vi "Meas Write Record Header File.vi"(6 "samples count":i64, 7 "corrections":T1 {"transducers"."channels"."Phase index" min=1 step=1}, 8 "error in":errorcluster, 9 "adc session":T4={"niScope"={"channel cfg"=[], "sessions"=[], "multi cards"=FALSE, "channels"=0, "type"=enum."n/a", "memory [B/chn]"=0, "ext. clock [Hz]"=0.0, "samples count"=0, "use streaming"=FALSE, "proc setup"={"packet size [smpl]"=0, "current timeout [s]"=0.0, "blk2blk timeout [s]"=0.0, "event time"=timestamp(0 s since 1904-01-01), "temp sampl T [s]"=0.0, "data queue"=refnum, "stop notifier"=refnum, "proc ref"=refnum}, "sample width [B]"=0, "ranges [V]"=[], "trigger setup"={"coupling"=1, "level [V]"=0.0, "slope"=0, "mode"=enum."Immediate"}, "fs [Hz]"=0.0, "bitres [bit]"=0}, "3458A"={"channels"=[], "sync unit"={"VISA"="", "type"=enum."Picotest U6200A"}, "awg unit"={"type"=enum."Agilent 331xxA to 332xxA", "VISA"="", "enable 10MHz ref"=FALSE}, "sync mode"=enum."MASTER-SLAVE, MASTER clocked by TIMER", "streaming mode"=FALSE, "idn mode"=enum."Auto", "sampling mode"=enum."DCV", "Ts [s]"=0.0, "sample memory [B]"=0, "proc setup"={"channel id"=0, "packet size [smpl]"=0, "current timeout [s]"=0.0, "blk2blk timeout [s]"=0.0, "event time"=timestamp(0 s since 1904-01-01), "stop notifier"=refnum, "data queues"=[], "proc refs"=[], "bus semaphore"=refnum}, "sample size [B]"=0, "sample count"=0, "aux data"={"channel id"=0, "valid?"=[], "gain [V]"=[], "timestamp [s]"=[], "Ts [s]"=0.0, "abs timestamp"=timestamp(0 s since 1904-01-01), "t [deg C]"=[]}, "ranges [V]"=[], "aperture [s]"=0.0, "LEVEL trigger"={"edge"=enum."POS", "level [V]"=0.0, "coupling"=enum."DC"}, "trigger mode"=enum."AUTO", "measure temp.?"=FALSE, "disp mesages"=[], "shared bus?"=FALSE, "disable display?"=FALSE, "aper mode"=enum."Manual", "aper rules"=[]}, "dsdll"={"dsdll"={"dsdll path"=path "", "dsdll handle"=[], "output devices"=[], "capture devices"=[]}, "channels"=0, "device id"=0, "channel idns"=[], "proc setup"={"packet size [smpl]"=0, "current timeout [s]"=0.0, "blk2blk timeout [s]"=0.0, "event time"=timestamp(0 s since 1904-01-01), "data queue"=refnum, "stop notifier"=refnum, "proc ref"=refnum}, "samples count"=0, "fs [Hz]"=0.0}, "type"=enum."niScope", "channel idn str"=[], "aux instr idn str"=[], "modified?"=FALSE, "simadc"={"channels"=[], "range [V]"=0.0, "Ts step [s]"=0.0, "time [s]"=0.0, "fs [Hz]"=0.0, "count"=0, "smpl offset"=0, "set count"=0, "bit res"=0}, "force rst?"=FALSE, "exit mode"=enum."Immediate reset", "exit dly"=0.0, "exit tmr"=timestamp(0 s since 1904-01-01), "busy?"=FALSE, "accessed?"=FALSE, "QuADC session"={"channel cfg"=[], "sessions"=[], "multi cards"=FALSE, "channels"=0, "type"=enum."n/a", "memory [B/chn]"=0, "ext. clock [Hz]"=0.0, "samples count"=0, "use streaming"=FALSE, "proc setup"={"packet size [smpl]"=0, "current timeout [s]"=0.0, "blk2blk timeout [s]"=0.0, "event time"=timestamp(0 s since 1904-01-01), "temp sampl T [s]"=0.0, "data queue"=refnum, "stop notifier"=refnum, "proc ref"=refnum}, "sample width [B]"=0, "ranges [V]"=[], "trigger setup"={"coupling"=1, "level [V]"=0.0, "slope"=0, "mode"=enum."Immediate"}, "fs [Hz]"=0.0, "bitres [bit]"=0}} {"QuADC session"."trigger setup"."level [V]" format="%.2f"; "QuADC session"."trigger setup"."coupling" items=["AC"=0, "DC"=1, "HF Reject"=3, "LF Reject"=4, "AC Plus HF Reject"=1001]; "QuADC session"."channel cfg"."Clock fr. (Hz)" min=0.0 format="%#_9p"; "QuADC session"."channel cfg"."Number of JJ" min=1; "QuADC session"."channel cfg"."Range [Vpk]" min=0.0; "QuADC session"."channel cfg"."Channel" min=0; "3458A"."channels"."Range [Vpk]" min=0.0; "niScope"."trigger setup"."level [V]" format="%.2f"; "niScope"."trigger setup"."coupling" items=["AC"=0, "DC"=1, "HF Reject"=3, "LF Reject"=4, "AC Plus HF Reject"=1001]; "niScope"."channel cfg"."Range [Vpk]" min=0.0; "niScope"."channel cfg"."Channel" min=0}, 10 "aux data":T53, 11 "sequence item":T49) -> (0 "error out":errorcluster)   [LabVIEW 2013]
doc: "Write logged temperature data to the samples MAT file. It will write the data even if they are empty."
uses:
  adc/ADC Aux Data.ctl
  Meas Sequence Item.ctl
  Meas Sampling Configuration.ctl
  adc/ADC Trig Config.ctl
  adc/ADC Trig Mode Source.ctl
  adc/ADC Trig Coupling.ctl
  adc/ADC Trig Slope.ctl
  processing/QWTB/Meas Proc QWTB Algorithm Parameter Data.ctl
  adc/ADC Session.ctl
  drivers/niScope/niScope Session.ctl
  drivers/niScope/niScope Virtual Channel Config.ctl
  drivers/niScope/niScope Virtual Channel Mode.ctl
  drivers/niScope/niScope Virtual Channel Input Z.ctl
  drivers/niScope/niScope Virtual Channel Coupling.ctl
  drivers/niScope/niScope Type.ctl
  drivers/niScope/niScope Digitizing Process Options.ctl
  drivers/niScope/niScope Data Packet.ctl
  drivers/niScope/niScope Trigger Setup.ctl
  <instrlib>/niScope/Controls/niScope trigger coupling.ctl
  <instrlib>/niScope/Controls/niScope trigger slope.ctl
  drivers/DMM/3458A Digitizer Session.ctl
  drivers/DMM/3458A Virtual Channel Config.ctl
  drivers/Counter/Counter Session.ctl
  drivers/Counter/Counter Type.ctl
  drivers/AWG/AWG Session.ctl
  drivers/AWG/AWG Type.ctl
  drivers/DMM/3458A Sync Mode.ctl
  drivers/DMM/3458A Idn Mode.ctl
  drivers/DMM/3458A Digitizing Low Levels/Configure/Sampling Mode.ctl
  drivers/DMM/3458A Digitizing Process Options.ctl
  drivers/DMM/3458A Data Packet.ctl
  drivers/DMM/3458A Aux Record Data.ctl
  drivers/DMM/3458A Digitizing Low Levels/Configure/Level Setup.ctl
  drivers/DMM/3458A Digitizing Low Levels/Configure/First Sample Trigger.ctl
  drivers/DMM/3458A Aperture Selection Mode.ctl
  drivers/dsdll/DSDLL Session.ctl
  drivers/dsdll/dsdll.lvlibp/dsdll_instance.ctl
  drivers/dsdll/dsdll.lvlibp/dsdll_device_record.ctl
  drivers/dsdll/DSDLL Process Config.ctl
  drivers/dsdll/DSDLL Data Packet.ctl
  adc/ADC Type.ctl
  drivers/simulated_adc/SimAdc Config.ctl
  drivers/simulated_adc/SimAdc Channel Cfg.ctl
  adc/ADC On Close Action.ctl
  drivers/Quatsch_driver/QuADCDriver/QuADC Session.ctl
  drivers/Quatsch_driver/QuADCDriver/QuADC Virtual Channel Config.ctl
  drivers/Quatsch_driver/QuADCDriver/QuADC Virtual Channel Mode.ctl
  drivers/Quatsch_driver/QuADCDriver/QuADC Virtual Channel Input Z.ctl
  drivers/Quatsch_driver/QuADCDriver/QuADC Virtual Channel Coupling.ctl
  drivers/Quatsch_driver/QuADCDriver/QuADC Type.ctl
  drivers/Quatsch_driver/QuADCDriver/QuADC Digitizing Process Options.ctl
  drivers/Quatsch_driver/QuADCDriver/QuADC Data Packet.ctl
  drivers/Quatsch_driver/QuADCDriver/QuADC Trigger Setup.ctl
  Corrections/Corr Setup.ctl
  Corrections/Corr Tranducer Item.ctl
  Corrections/Corr Digitizers.ctl
  <vilib>/Analysis/baseanly.llb/Mean (DBL).vi
  octave/infolib.lvlibp/Private/Add matrix polymorph parts/1D String.vi
  octave/infolib.lvlibp/Private/Add key polymorph parts/I64.vi
  octave/infolib.lvlibp/Private/Add key polymorph parts/String.vi
  octave/infolib.lvlibp/Private/Add key polymorph parts/Boolean.vi
  octave/infolib.lvlibp/Private/Get key polymorph parts/GetI64.vi
  octave/infolib.lvlibp/Private/Add key polymorph parts/EXT.vi
  octave/infolib.lvlibp/Private/Add matrix polymorph parts/2D EXT.vi
  octave/infolib.lvlibp/Private/Add matrix polymorph parts/2D String.vi
  octave/infolib.lvlibp
  <vilib>/Analysis/NI_AALBase.lvlib
  drivers/niScope/niScope Virtual Digitizer.lvlib
  drivers/DMM/3458A Virtual Digitizer.lvlib
  drivers/Counter/Counter.lvlib
  drivers/AWG/AWG.lvlib
  drivers/DMM/3458A Digitizing Low Levels/3458A Digitizing Low Levels.lvlib
  drivers/dsdll/dsdll.lvlibp
  drivers/dsdll/DSDLL Virtual Digitizer.lvlib
  drivers/Quatsch_driver/QuADCDriver/QuADC Virtual Digitizer.lvlib
panel:
  in  "coupling":T46
  in  "slope":T47
  in  "source":T48
  # "ADC:"
  # "IP Address"
  # "."
  # "."
  # "."
  # ":"
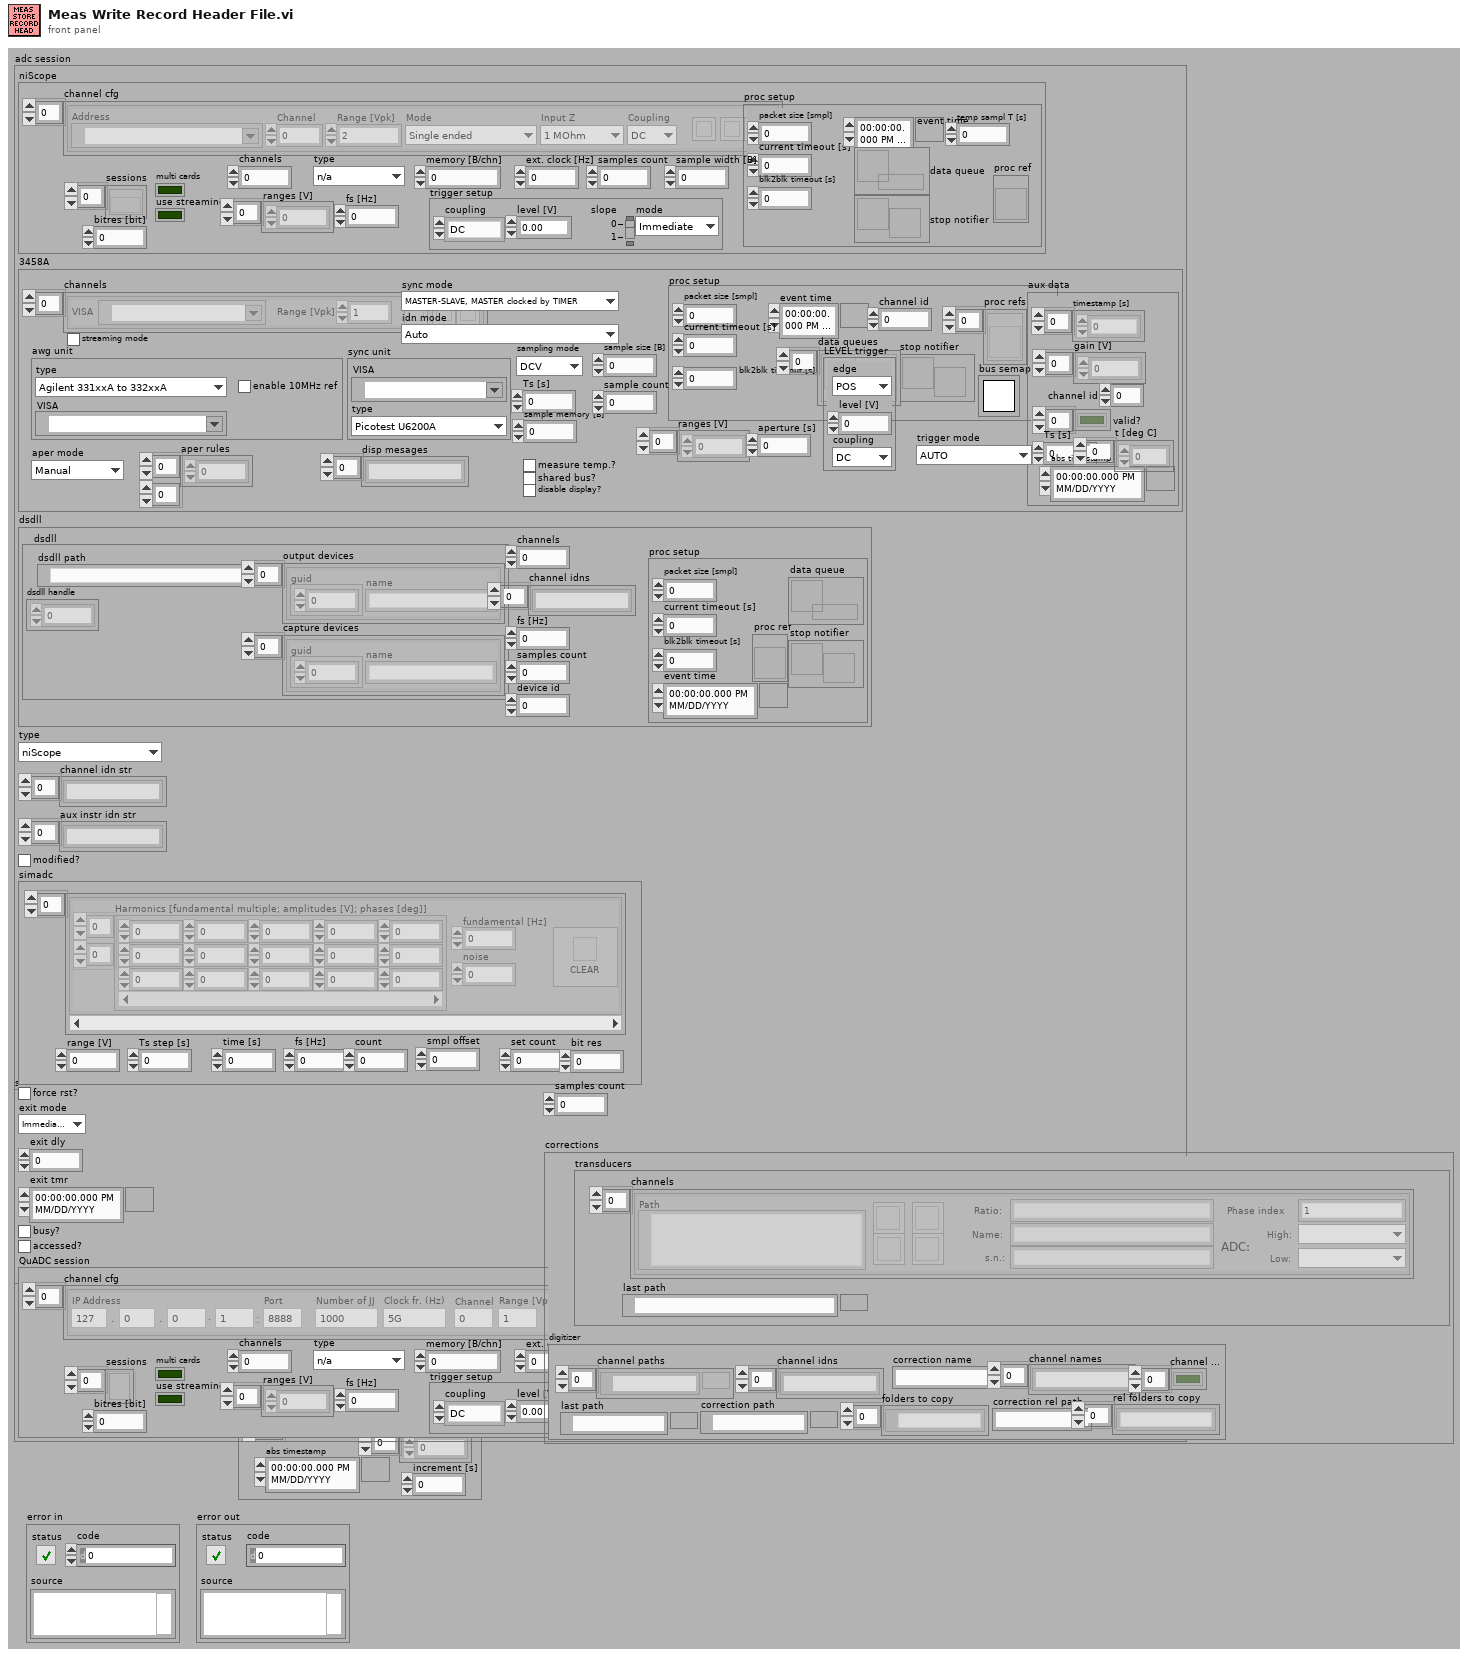
[diagram p1: front panel]
types:
  T1 = typedef "Corr Setup.ctl" = cluster{"transducers":cluster{"channels":T2[], "last path":path}, "digitizer":T3}
  T2 = typedef "Corr Tranducer Item.ctl" = cluster{"Path":path, "Ratio:":string, "Name:":string, "btn rem":bool, "btn up":bool, "btn down":bool, "s.n.:":string, "btn open":bool, "ratio o/i":dbl, "chn hi":u16, "chn lo":u16, "Phase index":i32}
  T3 = typedef "Corr Digitizers.ctl" = cluster{"last path":path, "channel paths":path[], "channel idns":string[], "correction name":string, "channel names":string[], "folders to copy":path[], "channel valid":bool[], "correction path":path, "correction rel path":string, "rel folders to copy":string[]}
  T4 = typedef "ADC Session.ctl" = cluster{"niScope":T5, "3458A":T15, "dsdll":T30, "type":T34, "channel idn str":string[], "aux instr idn str":string[], "modified?":bool, "simadc":T35, "force rst?":bool, "exit mode":T37, "exit dly":dbl, "exit tmr":timestamp, "busy?":bool, "accessed?":bool, "QuADC session":T38}
  T5 = typedef "niScope Virtual Digitizer.lvlib/niScope Session.ctl" = cluster{"channel cfg":T6[], "sessions":refnum<k20>[], "multi cards":bool, "channels":i32, "type":T10, "memory [B/chn]":i32, "ext. clock [Hz]":dbl, "samples count":i64, "use streaming":bool, "proc setup":T11, "sample width [B]":i32, "ranges [V]":dbl[], "trigger setup":T12, "fs [Hz]":dbl, "bitres [bit]":i32}
  T6 = typedef "niScope Virtual Digitizer.lvlib/niScope Virtual Channel Config.ctl" = cluster{"Address":refnum<k15>, "Channel":i32, "Mode":T7, "Input Z":T8, "Coupling":T9, "Range [Vpk]":dbl, "btn clr":bool, "btn up":bool, "btn down":bool}
  T7 = typedef "niScope Virtual Digitizer.lvlib/niScope Virtual Channel Mode.ctl" = enum16{"Single ended", "Unbal. differential", "Differential"}
  T8 = typedef "niScope Virtual Digitizer.lvlib/niScope Virtual Channel Input Z.ctl" = enum16{"1 MOhm", "50 Ohm"}
  T9 = typedef "niScope Virtual Digitizer.lvlib/niScope Virtual Channel Coupling.ctl" = enum16{"AC", "DC", "GND"}
  T10 = typedef "niScope Virtual Digitizer.lvlib/niScope Type.ctl" = enum16{"n/a", "5922"}
  T11 = typedef "niScope Virtual Digitizer.lvlib/niScope Digitizing Process Options.ctl" = cluster{"packet size [smpl]":i64, "current timeout [s]":dbl, "blk2blk timeout [s]":dbl, "event time":timestamp, "temp sampl T [s]":dbl, "data queue":refnum<queue>, "stop notifier":refnum<notifier>, "proc ref":refnum<vi>}
  T12 = typedef "niScope Virtual Digitizer.lvlib/niScope Trigger Setup.ctl" = cluster{"coupling":T13, "level [V]":dbl, "slope":T14, "mode":enum16{"Immediate", "External", "Level"}}
  T13 = typedef "niScope trigger coupling.ctl" = u16
  T14 = typedef "niScope trigger slope.ctl" = i32
  T15 = typedef "3458A Virtual Digitizer.lvlib/3458A Digitizer Session.ctl" = cluster{"channels":T16[], "sync unit":T17, "awg unit":T19, "sync mode":T21, "streaming mode":bool, "idn mode":T22, "sampling mode":T23, "Ts [s]":dbl, "sample memory [B]":i32, "proc setup":T24, "sample size [B]":i32, "sample count":i32, "aux data":T26, "ranges [V]":dbl[], "aperture [s]":dbl, "LEVEL trigger":T27, "trigger mode":T28, "measure temp.?":bool, "disp mesages":string[], "shared bus?":bool, "disable display?":bool, "aper mode":T29, "aper rules":dbl[][]}
  T16 = typedef "3458A Virtual Digitizer.lvlib/3458A Virtual Channel Config.ctl" = cluster{"VISA":refnum<visa-resource-name>, "Range [Vpk]":dbl, "btn clr":bool, "btn up":bool, "btn down":bool}
  T17 = typedef "Counter.lvlib/Counter Session.ctl" = cluster{"VISA":refnum<visa-resource-name>, "type":T18}
  T18 = typedef "Counter.lvlib/Counter Type.ctl" = enum16{"Picotest U6200A", "dummy"}
  T19 = typedef "AWG.lvlib/AWG Session.ctl" = cluster{"type":T20, "VISA":refnum<visa-resource-name>, "enable 10MHz ref":bool}
  T20 = typedef "AWG.lvlib/AWG Type.ctl" = enum16{"Agilent 331xxA to 332xxA", "Agilent 335xxA to 336xxA", "Tektronix AFG3101C", "dummy"}
  T21 = typedef "3458A Virtual Digitizer.lvlib/3458A Sync Mode.ctl" = enum16{"MASTER-SLAVE, MASTER clocked by TIMER", "MASTER-SLAVE, MASTER clocked by AWG", "ALL clocked by AWG", "MASTER-SLAVE, ALL clocked by TIMER", "ALL clocked by AWG with DFLL"}
  T22 = typedef "3458A Virtual Digitizer.lvlib/3458A Idn Mode.ctl" = enum16{"Auto", "Sequential (chn A, chn B, ...)", "From calibration string"}
  T23 = typedef "3458A Virtual Digitizer.lvlib/3458A Digitizing Low Levels.lvlib/Sampling Mode.ctl" = enum16{"DCV", "DSDC", "DSAC"}
  T24 = typedef "3458A Virtual Digitizer.lvlib/3458A Digitizing Process Options.ctl" = cluster{"channel id":i32, "packet size [smpl]":i32, "current timeout [s]":dbl, "blk2blk timeout [s]":dbl, "event time":timestamp, "stop notifier":refnum<notifier>, "data queues":refnum<queue>[], "proc refs":refnum<vi>[], "bus semaphore":T25}
  T25 = typedef "Semaphore RefNum" = refnum<k1>
  T26 = typedef "3458A Virtual Digitizer.lvlib/3458A Aux Record Data.ctl" = cluster{"channel id":i32, "valid?":bool[], "gain [V]":dbl[], "timestamp [s]":dbl[], "Ts [s]":dbl, "abs timestamp":timestamp, "t [deg C]":dbl[]}
  T27 = typedef "3458A Virtual Digitizer.lvlib/3458A Digitizing Low Levels.lvlib/Level Setup.ctl" = cluster{"edge":enum16{"POS", "NEG"}, "level [V]":dbl, "coupling":enum16{"DC", "AC"}}
  T28 = typedef "3458A Virtual Digitizer.lvlib/3458A Digitizing Low Levels.lvlib/First Sample Trigger.ctl" = enum16{"AUTO", "EXT", "SYN", "SGL", "HOLD", "LEVEL"}
  T29 = typedef "3458A Virtual Digitizer.lvlib/3458A Aperture Selection Mode.ctl" = enum16{"Manual", "Maximum", "Table"}
  T30 = typedef "DSDLL Virtual Digitizer.lvlib/DSDLL Session.ctl" = cluster{"dsdll":T31, "channels":i32, "device id":i32, "channel idns":string[], "proc setup":T33, "samples count":i32, "fs [Hz]":dbl}
  T31 = typedef "dsdll.lvlibp/dsdll_instance.ctl" = cluster{"dsdll path":path, "dsdll handle":u8[], "output devices":T32[], "capture devices":T32[]}
  T32 = typedef "dsdll.lvlibp/dsdll_device_record.ctl" = cluster{"guid":u8[], "name":string}
  T33 = typedef "DSDLL Virtual Digitizer.lvlib/DSDLL Process Config.ctl" = cluster{"packet size [smpl]":i32, "current timeout [s]":dbl, "blk2blk timeout [s]":dbl, "event time":timestamp, "data queue":refnum<queue>, "stop notifier":refnum<notifier>, "proc ref":refnum<vi>}
  T34 = typedef "ADC Type.ctl" = enum16{"niScope", "3458A", "DirectSound DLL", "dummy", "QuADC"}
  T35 = typedef "SimAdc Config.ctl" = cluster{"channels":T36[], "range [V]":dbl, "Ts step [s]":dbl, "time [s]":dbl, "fs [Hz]":dbl, "count":i64, "smpl offset":i64, "set count":i64, "bit res":i32}
  T36 = typedef "SimAdc Channel Cfg.ctl" = cluster{"harmonics":dbl[][], "btn clear":bool, "noise":dbl, "fundamental [Hz]":dbl}
  T37 = typedef "ADC On Close Action.ctl" = enum16{"Immediate reset", "Delayed reset"}
  T38 = typedef "QuADC Virtual Digitizer.lvlib/QuADC Session.ctl" = cluster{"channel cfg":T39[], "sessions":refnum<k5>[], "multi cards":bool, "channels":i32, "type":T43, "memory [B/chn]":i32, "ext. clock [Hz]":dbl, "samples count":i64, "use streaming":bool, "proc setup":T44, "sample width [B]":i32, "ranges [V]":dbl[], "trigger setup":T45, "fs [Hz]":dbl, "bitres [bit]":i32}
  T39 = typedef "QuADC Virtual Digitizer.lvlib/QuADC Virtual Channel Config.ctl" = cluster{"Channel":i32, "Mode":T40, "Input Z":T41, "Coupling":T42, "Range [Vpk]":dbl, "btn clr":bool, "btn up":bool, "btn down":bool, "IP address A":u8, "IP address B":u8, "IP address C":u8, "IP address D":u8, "Port":u16, "Number of JJ":u32, "Clock fr. (Hz)":dbl}
  T40 = typedef "QuADC Virtual Digitizer.lvlib/QuADC Virtual Channel Mode.ctl" = enum16{"Single ended", "Unbal. differential", "Differential"}
  T41 = typedef "QuADC Virtual Digitizer.lvlib/QuADC Virtual Channel Input Z.ctl" = enum16{"1 MOhm", "50 Ohm"}
  T42 = typedef "QuADC Virtual Digitizer.lvlib/QuADC Virtual Channel Coupling.ctl" = enum16{"AC", "DC", "GND"}
  T43 = typedef "QuADC Virtual Digitizer.lvlib/QuADC Type.ctl" = enum16{"n/a", "v1"}
  T44 = typedef "QuADC Virtual Digitizer.lvlib/QuADC Digitizing Process Options.ctl" = cluster{"packet size [smpl]":i64, "current timeout [s]":dbl, "blk2blk timeout [s]":dbl, "event time":timestamp, "temp sampl T [s]":dbl, "data queue":refnum<queue>, "stop notifier":refnum<notifier>, "proc ref":refnum<vi>}
  T45 = typedef "QuADC Virtual Digitizer.lvlib/QuADC Trigger Setup.ctl" = cluster{"coupling":T13, "level [V]":dbl, "slope":T14, "mode":enum16{"Immediate", "External", "Level"}}
  T46 = typedef "ADC Trig Coupling.ctl" = enum16{"DC", "AC"}
  T47 = typedef "ADC Trig Slope.ctl" = enum16{"POS", "NEG"}
  T48 = typedef "ADC Trig Mode Source.ctl" = enum16{"Immediate", "External", "Level"}
  T49 = typedef "Meas Sequence Item.ctl" = cluster{"config":T50, "data file path":path, "header file path":path, "group id":i32, "average id":i32, "group done?":bool, "adc modified?":bool, "source modified?":bool, "progress [%]":dbl, "groups cnt":i32, "average cnt":i32, "data file relative path":string, "meas root path":path, "calculate?":bool}
  T50 = typedef "Meas Sampling Configuration.ctl" = cluster{"fs [Hz]":dbl, "count [smpl]":i64, "aperture [s]":dbl, "trigger":T51, "ranges [Vpk]":dbl[], "QWTB parameters":T52[]}
  T51 = typedef "ADC Trig Config.ctl" = cluster{"source":T48, "level [V]":dbl, "coupling":T46, "slope":T47}
  T52 = typedef "Meas Proc QWTB Algorithm Parameter Data.ctl" = cluster{"name":string, "numerics":dbl[], "strings":string[]}
  T53 = typedef "ADC Aux Data.ctl" = cluster{"offset [V]":dbl[], "gain [V]":dbl[], "time stamp [s]":dbl[], "increment [s]":dbl, "T smpl":i64[], "T [deg C]":dbl[][], "valid?":bool, "abs timestamp":timestamp}
  T54 = typedef "ADC Capabilities.ctl" = cluster{"max samples count":i64, "max fs [Hz]":ext, "min fs [Hz]":ext, "Ts step [s]":ext, "max Ts [s]":ext, "min Ts [s]":ext, "allows streaming?":bool, "streaming on?":bool, "has level trig?":bool, "has ext trig?":bool, "has aperture?":bool, "aper min [s]":dbl, "aper max [s]":dbl, "channels count":i32, "has ranges?":bool, "has temperature?":bool, "has temperature log?":bool, "has selfcal?":bool, "fs step [Hz]":ext, "smpl rate step mode":T55}
  T55 = typedef "ADC Sampling Rate Step Mode.ctl" = enum16{"const period", "const frequency"}
  T56 = typedef "ADC Attribute.ctl" = cluster{"name":string, "value":string[], "is constant per group":bool}
  T57 = typedef "ADC Current Configuration.ctl" = cluster{"count [smpl]":i64, "channels count":i32, "fs [Hz]":dbl, "ranges [V]":dbl[], "trigger":T51, "ext freq. locked?":bool, "streaming on?":bool, "is int16?":bool, "bitres":i32}
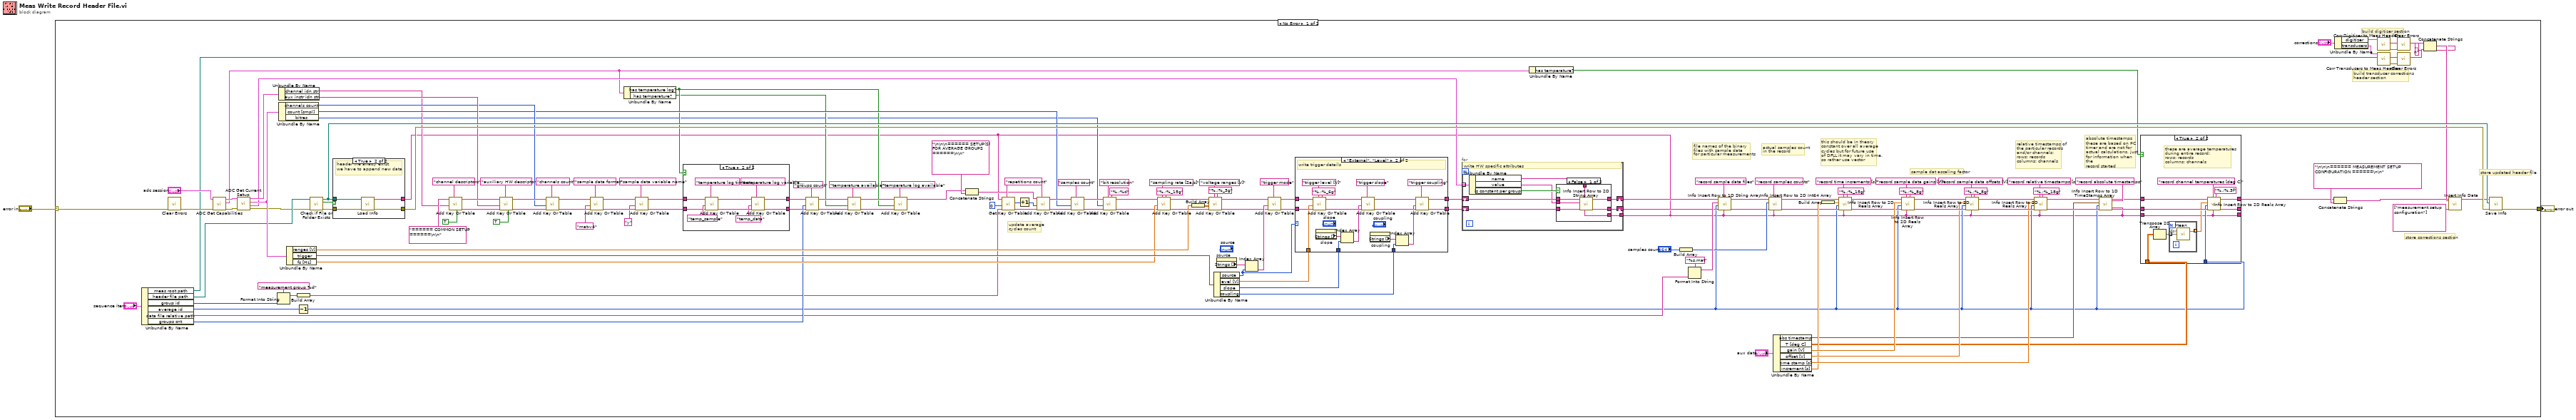
[diagram p0: block diagram]
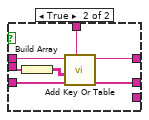
[diagram p4: hidden frame]
diagram:
  n1 = case shown="No Error" "error in" {
    selector: "error in" -> [w100 w237]
    tunnel: [w134 w237] -> w2
    frame No Error {
      w132 = "repetitions count" ("key description")
      # "store corrections section"
      # "build digitizer section"
      # "build transducer corrections\nheader section"
      # "actual samples count\nin the record"
      # "absolute timestamps\nthese are based on PC\ntimer and are not for \nactual calculations, just\nfor information when the\nrecord started"
      # "file names of the binary\nfiles with sample data\nfor particular measurements"
      # "relative timestamps of\nthe particular records\nand/or channels:\nrows: records\ncolumns: channels"
      # "sample dat ascaling factor"
      # "this should be in theory\nconstant over all average\ncycles but for future use\nof DFLL it may vary in time,\nso rather use vector"
      # "update average\ncycles count"
      # "store updated header file"
      n2 = Unbundle By Name("sequence item") -> ("meas root path"=w27:path, "header file path"=w34:path, "group id"=w47:i32, "average id"=w127:i32, "data file relative path"=w33:string, "groups cnt"=w46:i32)
      n3 = call <vilib>:"Clear Errors.vi"("error in (no error)"=w100) -> ("error out"=w76:errorcluster)  [unwired: 6 in]
      n4 = call "ADC Get Capabilities.vi"("error in"=w76, "adc session in"="adc session") -> ("error out"=w77:errorcluster, "capabilities"=w51:T54, "adc session out"=w74:T4)  [unwired: 7 in]
      n5 = call "ADC Get Current Setup.vi"("error in"=w77, "adc session in"=w74) -> ("error out"=w21:errorcluster, "device specific attributes"=w80:T56[], "common attributes"=w84:T57, "adc session out"=w110:T4)  [unwired: 6 in]
      n6 = Format Into String(format string="measurement group %d", w47) -> (resulting string=w112:string)  [unwired: 2 in, 1 out]
      n7 = Unbundle By Name(w110) -> ("channel idn str"=w14:string[], "aux instr idn str"=w106:string[])
      n8 = Unbundle By Name(w84) -> ("channels count"=w90:i32, "count [smpl]"=w58:i64, "bitres"=w5:i32)
      n9 = Unbundle By Name(w84) -> ("ranges [V]"=w83:dbl[], "trigger"=w82:T51, "fs [Hz]"=w81:dbl)
      n10 = Build Array(w112) -> (w22:string[])
      n11 = Decrement(x=w127) -> (x-1=w23:i32)
      n12 = call <vilib>:"Check if File or Folder Exists.vi"("error in (no error)"=w21, "path"=w34) -> ("error out"=w157:errorcluster, "file or folder exists?"=w158:bool, "dup path"=w136:path)  [unwired: 7 in]
      n13 = case shown="True" w158 {
        tunnel: w157 -> [w232 w236]
        tunnel: w136 -> [_ w235]
        tunnel: [_ w234] -> w4
        tunnel: [w232 w233] -> w135
        frame False {
          # "no header file exit\nstart new one"
        }
        frame True {
          # "header file alrady exist\nwe have to append new data"
          n14 = call "Load Info.vi"("error in"=w236, "filename"=w235) -> ("error out"=w233:errorcluster, "info data"=w234:string)  [unwired: 8 in]
        }
      }
      n15 = call-poly "Add Key Or Table.vi"("column vector (F)"=TRUE, "key description"="channel descriptors", "string"=w14, "info data"="====== COMMON SETUP ======\n\n" ("string")) -> ("sections out"=w109:string[], "info data out"=w108:string)  [unwired: 6 in]
      n16 = call-poly "Add Key Or Table.vi"("column vector (F)"=TRUE, "key description"="auxiliary HW descriptors", "sections"=w109, "string"=w106, "info data"=w108) -> ("sections out"=w103:string[], "info data out"=w102:string)  [unwired: 5 in]
      n17 = call-poly "Add Key Or Table.vi"("key description"="channels count", "sections"=w103, "numeric"=w90, "info data"=w102) -> ("sections out"=w98:string[], "info data out"=w97:string)  [unwired: 6 in]
      n18 = call-poly "Add Key Or Table.vi"("key description"="sample data format", "sections"=w98, "string"="mat-v4" ("multi-line string"), "info data"=w97) -> ("sections out"=w57:string[], "info data out"=w56:string)  [unwired: 6 in]
      n19 = Unbundle By Name(w51) -> ("has temperature log?"=w36:bool, "has temperature?"=w35:bool)
      n20 = call-poly "Add Key Or Table.vi"("key description"="sample data variable name", "sections"=w57, "string"="y", "info data"=w56) -> ("sections out"=w53:string[], "info data out"=w52:string)  [unwired: 6 in]
      n21 = case shown="True" w36 {
        tunnel: w53 -> [w160 w169]
        tunnel: w52 -> [w161 w168]
        tunnel: [w161 w164] -> w49
        tunnel: [w160 w162] -> w50
        frame False {
        }
        frame True {
          n22 = call-poly "Add Key Or Table.vi"("key description"="temperature log time stamp variable name", "sections"=w169, "string"="temp_sample", "info data"=w168) -> ("sections out"=w166:string[], "info data out"=w163:string)  [unwired: 6 in]
          n23 = call-poly "Add Key Or Table.vi"("key description"="temperature log variable name", "sections"=w166, "string"="temp_data", "info data"=w163) -> ("sections out"=w162:string[], "info data out"=w164:string)  [unwired: 6 in]
        }
      }
      n24 = call-poly "Add Key Or Table.vi"("key description"="groups count", "sections"=w50, "numeric"=w46, "info data"=w49) -> ("sections out"=w40:string[], "info data out"=w37:string)  [unwired: 6 in]
      n25 = call-poly "Add Key Or Table.vi"("key description"="temperature available", "sections"=w40, "boolean"=w35, "info data"=w37) -> ("sections out"=w39:string[], "info data out"=w41:string)  [unwired: 6 in]
      n26 = call-poly "Add Key Or Table.vi"("key description"="temperature log available", "sections"=w39, "boolean"=w36, "info data"=w41) -> ("info data out"=w38:string)  [unwired: 6 in, 1 out]
      n27 = Concatenate Strings(w38, "\n\n\n====== SETUP(S) FOR AVERAGE GROUPS ======\n\n" ("string")) -> (w105:string)
      n28 = call-poly "Get Key Or Table.vi"("key description"=w132, "sections"=w22, "numeric"=i64 0, "info data"=w4) -> ("sections out"=w133:string[], "value"=w131:i64)  [unwired: 4 in, 2 out]
      n29 = Increment(x=w131) -> (x+1=w130:i64)
      n30 = call-poly "Add Key Or Table.vi"("key description"=w132, "sections"=w133, "numeric"=w130, "info data"=w105) -> ("sections out"=w61:string[], "info data out"=w60:string)  [unwired: 6 in]
      n31 = call-poly "Add Key Or Table.vi"("key description"="samples count", "sections"=w61, "numeric"=w58, "info data"=w60) -> ("sections out"=w9:string[], "info data out"=w6:string)  [unwired: 6 in]
      n32 = call-poly "Add Key Or Table.vi"("format string (%_20d)"="%.;%d" ("format string (%_20f)"), "key description"="bit resolution", "sections"=w9, "numeric"=w5, "info data"=w6) -> ("sections out"=w8:string[], "info data out"=w7:string)  [unwired: 5 in]
      n33 = call-poly "Add Key Or Table.vi"("format string (%_20f)"="%.;%_15g", "key description"="sampling rate [Sa/s]", "sections"=w8, "numeric"=w81, "info data"=w7) -> ("sections out"=w86:string[], "info data out"=w85:string)  [unwired: 5 in]
      n34 = Build Array(w83) -> (w91:dbl[][])
      n35 = call-poly "Add Key Or Table.vi"("format string (%_20f)"="%.;%_3g", "key description"="voltage ranges [V]", "sections"=w86, "numeric"=w91, "info data"=w85) -> ("sections out"=w94:string[], "info data out"=w95:string)  [unwired: 5 in]
      n36 = Unbundle By Name(w82) -> ("source"=w118:T48, "level [V]"=w116:dbl, "slope"=w115:T47, "coupling"=w114:T46)
      n37 = property on="source" class="Enum (strict)"() -> ("Strings []"=w120:string[])  [unwired: 2 in, 2 out]
      n38 = Index Array(array=w120, index=w118) -> (element=w119:string)
      n39 = call-poly "Add Key Or Table.vi"("key description"="trigger mode", "sections"=w94, "string"=w119, "info data"=w95) -> ("sections out"=w117:string[], "info data out"=w113:string)  [unwired: 6 in]
      n40 = case shown="\"External\", \"Level\"" w118 {
        tunnel: w117 -> [w212 w231]
        tunnel: w116 -> [_ w228]
        tunnel: w115 -> [_ w224]
        tunnel: w114 -> [_ w219]
        tunnel: [w212 w215] -> w79
        tunnel: [w211 w214] -> w78
        tunnel: w113 -> [w211 w213]
        frame Default {
        }
        frame "External", "Level" {
          # "write trigger details"
          n41 = call-poly "Add Key Or Table.vi"("format string (%_20f)"="%.;%_6g", "key description"="trigger level [V]", "sections"=w231, "numeric"=w228, "info data"=w213) -> ("sections out"=w226:string[], "info data out"=w217:string)  [unwired: 5 in]
          n42 = property on="slope" class="Enum (strict)"() -> ("Strings []"=w225:string[])  [unwired: 2 in, 2 out]
          n43 = Index Array(array=w225, index=w224) -> (element=w223:string)
          n44 = call-poly "Add Key Or Table.vi"("key description"="trigger slope", "sections"=w226, "string"=w223, "info data"=w217) -> ("sections out"=w221:string[], "info data out"=w216:string)  [unwired: 6 in]
          n45 = property on="coupling" class="Enum (strict)"() -> ("Strings []"=w220:string[])  [unwired: 2 in, 2 out]
          n46 = Index Array(array=w220, index=w219) -> (element=w218:string)
          n47 = call-poly "Add Key Or Table.vi"("key description"="trigger coupling", "sections"=w221, "string"=w218, "info data"=w216) -> ("sections out"=w215:string[], "info data out"=w214:string)  [unwired: 6 in]
        }
      }
      n48 = for {
        tunnel: w80 -> [w196] mode=indexing
        shift-right: [w195] -> w44
        shift-left: w79 -> [w192]
        shift-right: [w194] -> w20
        shift-left: w78 -> [w193]
        tunnel: w4 -> [w188]
        # "write HW specific attributes"
        n49 = Unbundle By Name(w196) -> ("name"=w191:string, "value"=w189:string[], "is constant per group"=w190:bool)
        n50 = case shown="False" w190 {
          tunnel: [w202 w210] -> w195
          tunnel: [w201 w209] -> w194
          tunnel: w193 -> [w200 w208]
          tunnel: w192 -> [w203 w207]
          tunnel: w191 -> [w199 w206]
          tunnel: w189 -> [w198 w204]
          tunnel: w188 -> [w197 _]
          frame False {
            n51 = call "Info Insert Row to 2D String Array.vi"("source info data"=w197, "key description"=w199, "sections in"=w203, "row to insert"=w198, "info data in"=w200) -> ("sections out"=w202:string[], "info data out"=w201:string)  [unwired: 5 in]
          }
          frame True {
            n52 = Build Array(w204) -> (w205:string[][])
            n53 = call-poly "Add Key Or Table.vi"("key description"=w206, "sections"=w207, "string"=w205, "info data"=w208) -> ("sections out"=w210:string[], "info data out"=w209:string)  [unwired: 6 in]
          }
        }
      }
      n54 = Unbundle By Name(w51) -> ("has temperature?"=w68:bool)
      n55 = Build Array("samples count") -> (w87:i64[])
      n56 = Format Into String(format string="%s.mat", w33) -> (resulting string=w124:string)  [unwired: 2 in, 1 out]
      n57 = call "Info Insert Row to 1D String Array.vi"("source info data"=w4, "key description"="record sample data files", "sections in"=w44, "row index to insert"=w23, "string to insert"=w124, "info data in"=w20) -> ("sections out"=w62:string[], "info data out"=w65:string)  [unwired: 4 in]
      n58 = call "Info Insert Row to 2D Int64 Array.vi"("source info data"=w4, "key description"="record samples counts", "sections in"=w62, "row to insert"=w87, "info data in"=w65) -> ("sections out"=w63:string[], "info data out"=w64:string)  [unwired: 5 in]
      n59 = Unbundle By Name("aux data") -> ("abs timestamp"=w66:timestamp, "T [deg C]"=w67:dbl[][], "gain [V]"=w154:dbl[], "offset [V]"=w148:dbl[], "time stamp [s]"=w143:dbl[], "increment [s]"=w138:dbl)
      n60 = Build Array(w138) -> (w137:dbl[])
      n61 = call "Info Insert Row to 2D Reals Array.vi"("format string (%_20f)"="%.;%_15g", "source info data"=w4, "key description"="record time increments [s]", "sections in"=w63, "row index to insert"=w23, "row to insert"=w137, "info data in"=w64) -> ("sections out"=w140:string[], "info data out"=w139:string)  [unwired: 3 in]
      n62 = call "Info Insert Row to 2D Reals Array.vi"("format string (%_20f)"="%.;%_8g", "source info data"=w4, "key description"="record sample data gains [V]", "sections in"=w140, "row index to insert"=w23, "row to insert"=w154, "info data in"=w139) -> ("sections out"=w150:string[], "info data out"=w149:string)  [unwired: 3 in]
      n63 = call "Info Insert Row to 2D Reals Array.vi"("format string (%_20f)"="%.;%_8g", "source info data"=w4, "key description"="record sample data offsets [V]", "sections in"=w150, "row index to insert"=w23, "row to insert"=w148, "info data in"=w149) -> ("sections out"=w145:string[], "info data out"=w144:string)  [unwired: 3 in]
      n64 = call "Info Insert Row to 2D Reals Array.vi"("format string (%_20f)"="%.;%_18g", "source info data"=w4, "key description"="record relative timestamps [s]", "sections in"=w145, "row index to insert"=w23, "row to insert"=w143, "info data in"=w144) -> ("sections out"=w73:string[], "info data out"=w72:string)  [unwired: 3 in]
      n65 = call "Info Insert Row to 1D TimeStamps Array.vi"("source info data"=w4, "key description"="record absolute timestamps", "sections in"=w73, "row index to insert"=w23, "timestamp to insert"=w66, "info data in"=w72) -> ("sections out"=w70:string[], "info data out"=w69:string)  [unwired: 4 in]
      n66 = case shown="True" w68 {
        tunnel: w70 -> [w173 w185]
        tunnel: w23 -> [_ w183]
        tunnel: w4 -> [w172 w176]
        tunnel: w69 -> [w174 w182]
        tunnel: [w173 w181] -> _
        tunnel: [w174 w180] -> w3
        tunnel: [w172 w176] -> _
        tunnel: w67 -> [_ w178]
        frame False {
        }
        frame True {
          # "these are average temperatures\nduring entire record:\nrows: records\ncolumns: channels"
          n67 = Transpose 2D Array(2D array=w178) -> (transposed array=w175:dbl[][])
          n68 = for {
            tunnel: w175 -> [w187] mode=indexing
            tunnel: [w186] -> w177 mode=indexing
            n69 = call-poly <vilib>:"Mean.vi"("X"=w187) -> ("mean"=w186:dbl)  [unwired: 1 out]
          }
          n70 = call "Info Insert Row to 2D Reals Array.vi"("format string (%_20f)"="%.;%.3f", "source info data"=w176, "key description"="record channel temperatures [deg C]", "sections in"=w185, "row index to insert"=w183, "row to insert"=w177, "info data in"=w182) -> ("sections out"=w181:string[], "info data out"=w180:string)  [unwired: 3 in]
        }
      }
      n71 = Concatenate Strings(w3, "\n\n\n====== MEASUREMENT SETUP CONFIGURATION ======\n\n" ("string")) -> (w28:string)
      n72 = Unbundle By Name("corrections") -> ("digitizer"=w24:T3, "transducers"=w26:cluster{"channels":T2[], "last path":path})
      n73 = call "Corr Digitizer to Meas Header.vi"("digitizer in"=w24) -> ("error out"=w25:errorcluster, "info data out"=w18:string)  [unwired: 8 in, 1 out]
      n74 = call "Corr Transducers to Meas Header.vi"("measurement root path"=w27, "transducers in"=w26) -> ("error out"=w31:errorcluster, "info data out"=w16:string)  [unwired: 7 in, 1 out]
      n75 = call <vilib>:"Clear Errors.vi"("error in (no error)"=w25) -> ()  [unwired: 6 in, 1 out]
      n76 = call <vilib>:"Clear Errors.vi"("error in (no error)"=w31) -> ()  [unwired: 6 in, 1 out]
      n77 = Concatenate Strings(w18, "\n" ("string"), w16) -> (w17:string)
      n78 = call "Insert Info Data.vi"("info data to insert"=w17, "sections"=string[] ["measurement setup configuration"], "info data"=w28) -> ("info data out"=w19:string)  [unwired: 7 in, 1 out]
      n79 = call "Save Info.vi"("error in"=w135, "filename"=w136, "info data"=w19) -> ("error out"=w134:errorcluster)  [unwired: 8 in]
    }
    frame Error {
    }
  }
  "error out" <- w2
